vi "Ejercicio_17_Generacion_PWM.vi"() -> ()   [LabVIEW 2020]
panel:
  in  "Duty Cycle (%)":dbl=50.0
  out "Waveform Chart":dynamicdata(graph)
  in  "stop":bool
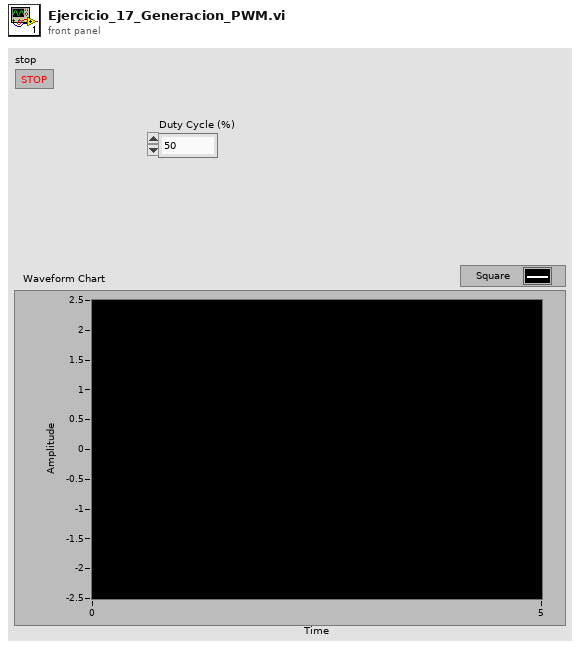
[diagram p1: front panel]
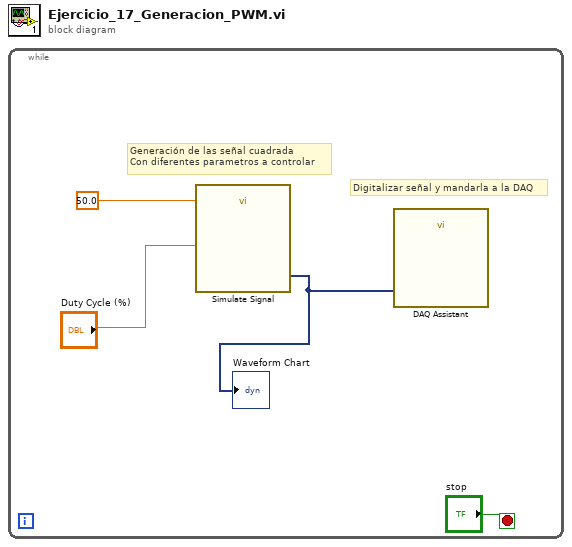
[diagram p0: block diagram]
diagram:
  n1 = while {
    stop <- "stop" stop-if-true
    # "Digitalizar señal y mandarla a la DAQ"
    # "Generación de las señal cuadrada\nCon diferentes parametros a controlar"
    n2 = call "Simulate Signal"("Duty Cycle (%)"="Duty Cycle (%)", "Frequency"=50.0) -> ("Square"=w2:dynamicdata)  [unwired: 12 in, 1 out]
    "Waveform Chart" <- w2
    n3 = call "DAQ Assistant"("data"=w2) -> ()  [unwired: 17 in, 2 out]
  }
